vi "systemXMLExpresssion.vi"(6 "xmlParser 1":string[](array[string]), 9 "index":i32, 10 "xmlParser 0":string[](array[string]), 11 "String":string) -> (2 "Numeric":i32, 3 "output array":string[](array[string]))   [LabVIEW 2018]
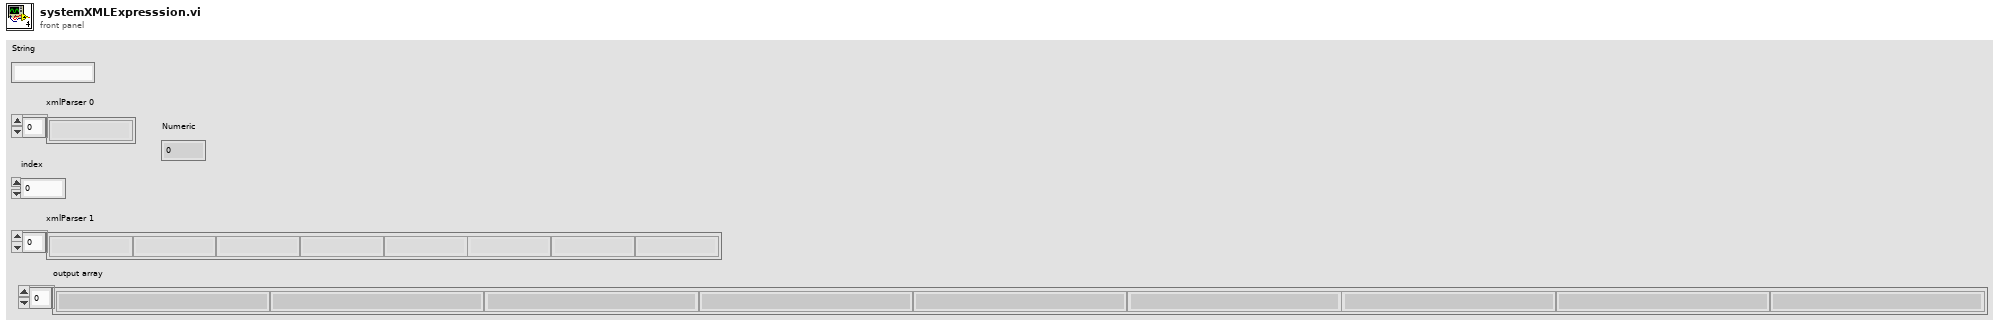
[diagram p1: front panel]
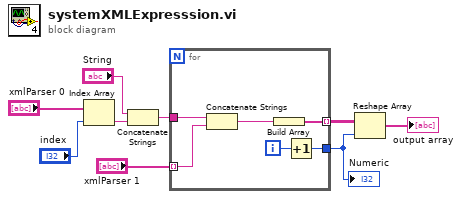
[diagram p0: block diagram]
diagram:
  n1 = Index Array(array="xmlParser 0", index="index") -> (element=w7:string)
  n2 = Concatenate Strings("String", w7) -> (w8:string)
  n3 = for {
    tunnel: "xmlParser 1" -> [w15] mode=indexing
    tunnel: [w13] -> w4 mode=indexing
    tunnel: w8 -> [w12]
    tunnel: [w10] -> w1
    i -> [w11]
    n4 = Concatenate Strings(w12, w15) -> (w14:string)
    n5 = Build Array(w14) -> (w13:string[])
    n6 = Increment(x=w11) -> (x+1=w10:i32)
  }
  "Numeric" <- w1
  n7 = Reshape Array(w4, w1) -> (→"output array":string[])
